vi "Read Harmonics to measure.vi"(11 "Harmonics in":refnum<class "Harmonics.lvclass">) -> (2 "Harmonics to measure":i32[](array[numeric]), 3 "Harmonics out":refnum<class "Harmonics.lvclass">)   [LabVIEW 2020, in "Harmonics.lvclass"]
uses:
  Harmonics.lvclass
  Harmonics.lvclass/Harmonics.ctl
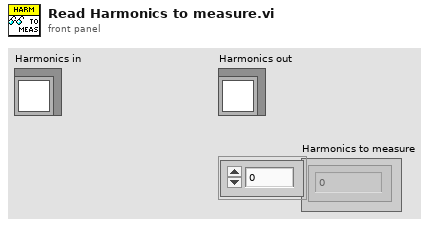
[diagram p1: front panel]
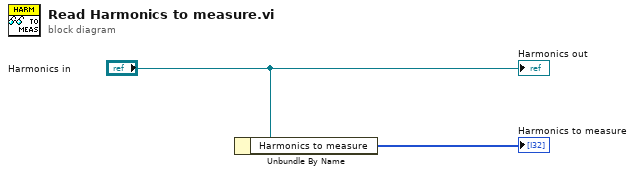
[diagram p0: block diagram]
diagram:
  n1 = Unbundle By Name("Harmonics in") -> ("Harmonics to measure"=→"Harmonics to measure":i32[])
  "Harmonics out" <- "Harmonics in"
